vi "can to speed.vi"(11 "Input can Array":string[][](array[string])) -> (1 "wyj nowe P":cluster{"8":sgl, "9":sgl, "10":sgl}, 2 "Napedy":T1, 3 "wyj nowe L":cluster{"8":sgl, "9":sgl, "10":sgl})   [LabVIEW 2015]
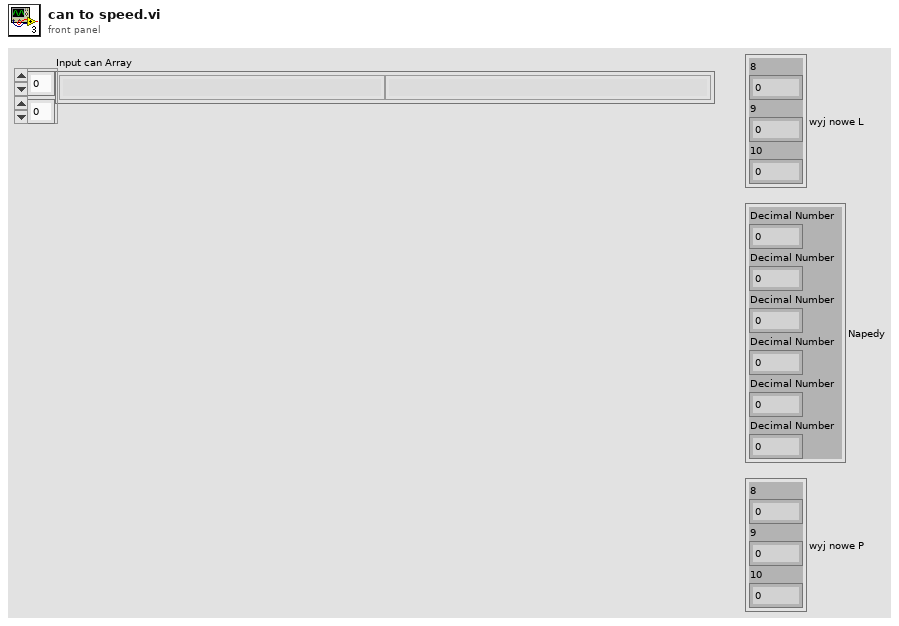
[diagram p1: front panel]
types:
  T1 = cluster{"Decimal Number":sgl, "Decimal Number":sgl, "Decimal Number":sgl, "Decimal Number":sgl, "Decimal Number":sgl, "Decimal Number":sgl}
  T2 = cluster{"Decimal Number":sgl, "Decimal Number":sgl, "Decimal Number":sgl}
  T3 = cluster{"Decimal Number":dbl, "Decimal Number":dbl, "Decimal Number":dbl, "Decimal Number":dbl, "Decimal Number":dbl, "Decimal Number":dbl}
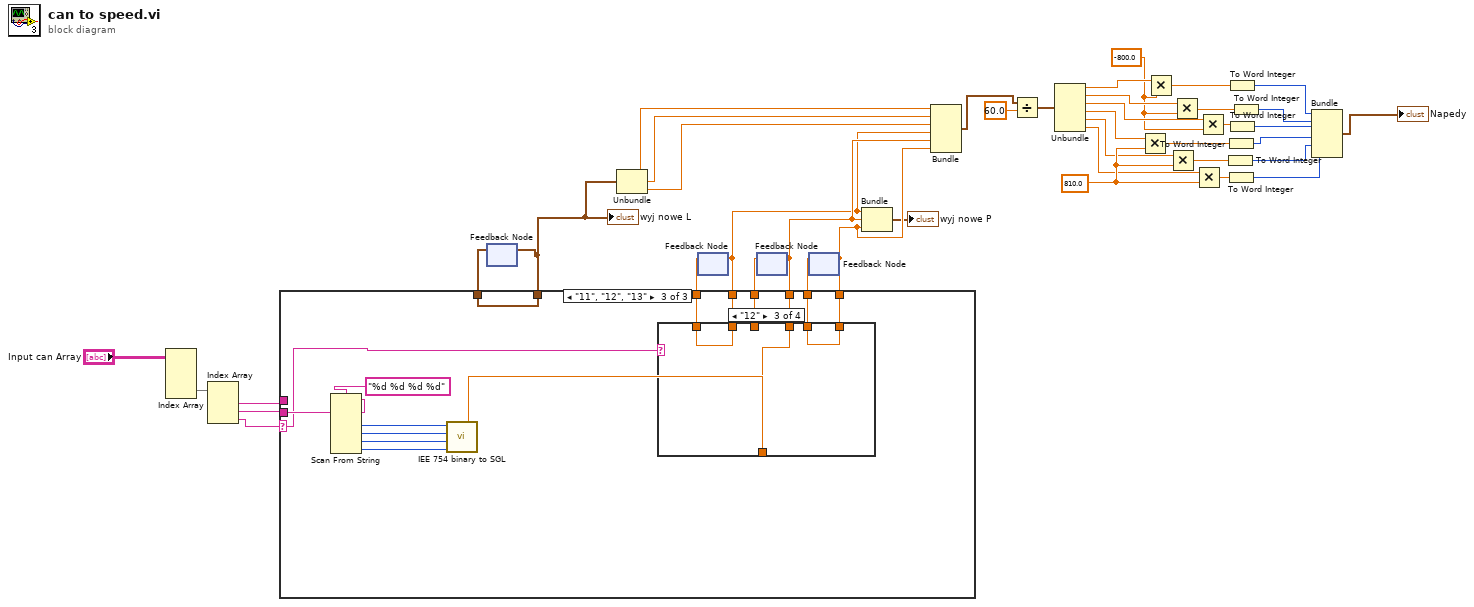
[diagram p0: block diagram]
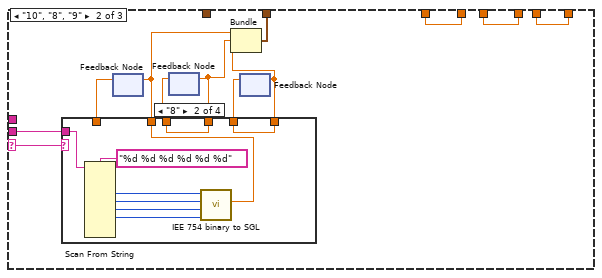
[diagram p3: hidden frame]
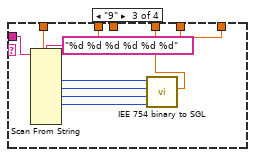
[diagram p5: hidden frame]
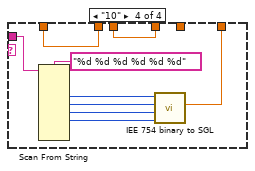
[diagram p6: hidden frame]
diagram:
  w14 = 810.0
  w15 = -800.0
  n1 = Index Array(array="Input can Array") -> (element #2=w26:string[])  [unwired: 4 in, 1 out]
  n2 = Index Array(array=w26) -> (element #1=w28:string, element #2=w27:string, element #3=w29:string)  [unwired: 3 in]
  n3 = feedback #1() -> (w34:T2)  [unwired: 1 in]
  n4 = feedback #2() -> (w33:sgl)  [unwired: 1 in]
  n5 = feedback #3() -> (w32:sgl)  [unwired: 1 in]
  n6 = feedback #4() -> (w31:sgl)  [unwired: 1 in]
  n7 = case shown="\"11\", \"12\", \"13\"" w29 {
    selector: w29 -> [_ w57 w90]
    tunnel: w27 -> [_ w46 w101]
    tunnel: w28 -> [_ _ _]
    tunnel: [w45 w56 w91] -> w39
    tunnel: w33 -> [w45 w56 w94]
    tunnel: [w44 w55 w92] -> w40
    tunnel: w32 -> [w44 w55 w95]
    tunnel: [w43 w54 w93] -> w41
    tunnel: w31 -> [w43 w54 w96]
    tunnel: [w42 w49 w88] -> w35
    tunnel: w34 -> [w42 _ w88]
    frame "False", Default {
    }
    frame "10", "8", "9" {
      n8 = feedback #5() -> (w53:sgl)  [unwired: 1 in]
      n9 = feedback #6() -> (w47:sgl)  [unwired: 1 in]
      n10 = feedback #7() -> (w48:sgl)  [unwired: 1 in]
      n11 = case shown="\"8\"" w57 {
        tunnel: [w58 w61 w78 w87] -> w52
        tunnel: [w60 w69 w72 w86] -> w51
        tunnel: [w59 w68 w70 w79] -> w50
        tunnel: w53 -> [w58 _ w78 w87]
        tunnel: w48 -> [w59 w68 w70 _]
        tunnel: w47 -> [w60 w69 _ w86]
        tunnel: w46 -> [_ w62 w71 w80]
        frame "False", Default {
        }
        frame "8" {
          n12 = Scan From String(format string="%d %d %d %d %d %d", input string=w62) -> (output 1=w64:i32, output 2=w65:i32, output 3=w66:i32, output 4=w67:i32)  [unwired: 10 in, 3 out]
          n13 = call "IEE 754 binary to SGL.vi"("Numeric"=w67, "Numeric 2"=w66, "Numeric 3"=w65, "Numeric 4"=w64) -> ("Decimal Number"=w61:sgl)  [unwired: 7 in]
        }
        frame "9" {
          n14 = Scan From String(format string="%d %d %d %d %d %d", input string=w71) -> (output 1=w74:i32, output 2=w75:i32, output 3=w76:i32, output 4=w77:i32)  [unwired: 10 in, 3 out]
          n15 = call "IEE 754 binary to SGL.vi"("Numeric"=w77, "Numeric 2"=w76, "Numeric 3"=w75, "Numeric 4"=w74) -> ("Decimal Number"=w72:sgl)  [unwired: 7 in]
        }
        frame "10" {
          n16 = Scan From String(format string="%d %d %d %d %d %d", input string=w80) -> (output 1=w82:i32, output 2=w83:i32, output 3=w84:i32, output 4=w85:i32)  [unwired: 10 in, 3 out]
          n17 = call "IEE 754 binary to SGL.vi"("Numeric"=w85, "Numeric 2"=w84, "Numeric 3"=w83, "Numeric 4"=w82) -> ("Decimal Number"=w79:sgl)  [unwired: 7 in]
        }
      }
      n18 = feedback-in #5(w52) -> ()
      n19 = feedback-in #6(w51) -> ()
      n20 = Bundle("Decimal Number"=w52, "Decimal Number"=w51, "Decimal Number"=w50) -> (w49:T2)  [unwired: 1 in]
      n21 = feedback-in #7(w50) -> ()
    }
    frame "11", "12", "13" {
      n22 = Scan From String(format string="%d %d %d %d", input string=w101) -> (output 1=w100:i32, output 2=w99:i32, output 3=w98:i32, output 4=w97:i32)  [unwired: 6 in, 3 out]
      n23 = call "IEE 754 binary to SGL.vi"("Numeric"=w97, "Numeric 2"=w98, "Numeric 3"=w99, "Numeric 4"=w100) -> ("Decimal Number"=w89:sgl)  [unwired: 7 in]
      n24 = case shown="\"12\"" w90 {
        tunnel: [w105 w108 w110 w113] -> w91
        tunnel: w89 -> [_ w108 w111 w114]
        tunnel: [w104 w107 w111 w112] -> w92
        tunnel: [w103 w106 w109 w114] -> w93
        tunnel: w94 -> [w105 _ w110 w113]
        tunnel: w95 -> [w104 w107 _ w112]
        tunnel: w96 -> [w103 w106 w109 _]
        frame "False", Default {
        }
        frame "11" {
        }
        frame "12" {
        }
        frame "13" {
        }
      }
    }
  }
  "wyj nowe L" <- w35
  n25 = feedback-in #1(w35) -> ()
  n26 = Unbundle(w35) -> ("Decimal Number"=w37:sgl, "Decimal Number"=w36:sgl, "Decimal Number"=w38:sgl)
  n27 = feedback-in #2(w39) -> ()
  n28 = feedback-in #3(w40) -> ()
  n29 = feedback-in #4(w41) -> ()
  n30 = Bundle("Decimal Number"=w39, "Decimal Number"=w40, "Decimal Number"=w41) -> (→"wyj nowe P":T2)  [unwired: 1 in]
  n31 = Bundle("Decimal Number"=w37, "Decimal Number"=w36, "Decimal Number"=w38, "Decimal Number"=w39, "Decimal Number"=w40, "Decimal Number"=w41) -> (w8:T1)  [unwired: 1 in]
  n32 = Divide(x=w8, y=60.0 ("mean")) -> (x/y=w9:T3)
  n33 = Unbundle(w9) -> ("Decimal Number"=w18:dbl, "Decimal Number"=w17:dbl, "Decimal Number"=w16:dbl, "Decimal Number"=w11:dbl, "Decimal Number"=w12:dbl, "Decimal Number"=w13:dbl)
  n34 = Multiply(x=w11, y=w14) -> (x*y=w19:dbl)
  n35 = Multiply(x=w18, y=w15) -> (x*y=w22:dbl)
  n36 = Multiply(x=w12, y=w14) -> (x*y=w20:dbl)
  n37 = Multiply(x=w17, y=w15) -> (x*y=w23:dbl)
  n38 = Multiply(x=w13, y=w14) -> (x*y=w21:dbl)
  n39 = Multiply(x=w16, y=w15) -> (x*y=w24:dbl)
  n40 = To Word Integer(number=w20) -> (16bit integer=w3:i16)
  n41 = To Word Integer(number=w19) -> (16bit integer=w4:i16)
  n42 = To Word Integer(number=w21) -> (16bit integer=w2:i16)
  n43 = To Word Integer(number=w22) -> (16bit integer=w7:i16)
  n44 = To Word Integer(number=w24) -> (16bit integer=w5:i16)
  n45 = To Word Integer(number=w23) -> (16bit integer=w6:i16)
  n46 = Bundle(w7, w6, w5, w4, w3, w2) -> (→"Napedy":cluster{i16, i16, i16, i16, i16, i16})  [unwired: 1 in]
